vi "Open Project.vi"(0 "path":path, 11 "error in":errorcluster) -> (4 "project ref":refnum<vi>, 15 "error out":errorcluster)   [LabVIEW 2021, in "G-Plugin Editor.lvlib"]
uses:
  G-Plugin Editor.lvlib
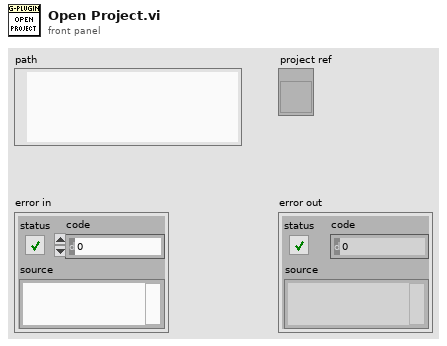
[diagram p1: front panel]
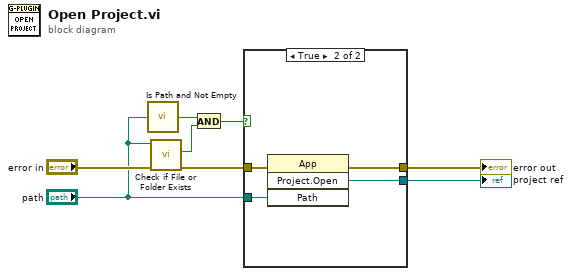
[diagram p0: block diagram]
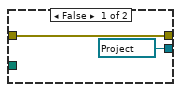
[diagram p2: hidden frame]
diagram:
  n1 = call <vilib>:"Is Path and Not Empty.vi"("path"="path") -> ("Is Path and Not Empty?"=w3:bool)  [unwired: 4 in]
  n2 = call <vilib>:"Check if File or Folder Exists.vi"("error in (no error)"="error in", "path"="path") -> ("error out"=w5:errorcluster, "file or folder exists?"=w2:bool)  [unwired: 7 in, 1 out]
  n3 = And(x=w3, y=w2) -> (x .and. y?=w1:bool)
  n4 = case shown="True" w1 {
    tunnel: [w10 w14] -> w7
    tunnel: [refnum<vi> refnum ("Project:Open") w13] -> w6
    tunnel: w5 -> [w10 w12]
    tunnel: "path" -> [_ w11]
    frame False {
    }
    frame True {
      n5 = invoke class="App" method="Project.Open"(error in=w12, "Path"=w11) -> (error out=w14:errorcluster, "Project:Open"=w13:refnum<vi>)  [unwired: 2 in, 2 out]
    }
  }
  "error out" <- w7
  "project ref" <- w6
